vi "instrument final.vi"() -> ()   [LabVIEW 2019]
panel:
  out "Mesaj corupt":bool
  out "String 2":string
  in  "String":string
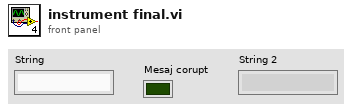
[diagram p1: front panel]
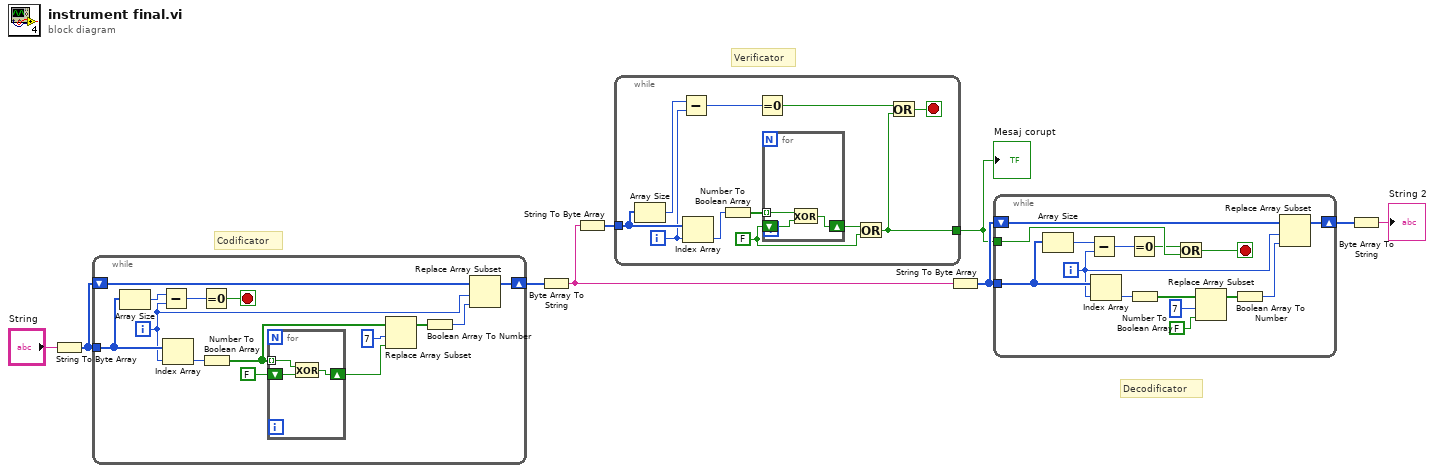
[diagram p0: block diagram]
diagram:
  # "Decodificator"
  # "Verificator"
  # "Codificator"
  n1 = String To Byte Array(string="String") -> (unsigned byte array=w5:u8[])
  n2 = while {
    tunnel: w5 -> [w23]
    shift-right: [w13] -> w4
    shift-left: w5 -> [w12]
    i -> [w11]
    stop <- w20 stop-if-true
    n3 = Array Size(array=w23) -> (size(s)=w22:i32)
    n4 = Subtract(x=w22, y=w11) -> (x-y=w21:i32)
    n5 = Index Array(array=w23, index=w11) -> (element=w15:u8)
    n6 = Equal To 0?(x=w21) -> (x = 0?=w20:bool)
    n7 = Number To Boolean Array(number=w15) -> (Boolean array=w17:bool[])
    n8 = for {
      tunnel: w17 -> [w24] mode=indexing
      shift-right: [w25] -> w18
      shift-left: FALSE -> [w26]
      n9 = Exclusive Or(1:w26, 2:w24) -> (0:w25:bool)
    }
    n10 = Replace Array Subset(array=w17, new element=w18, index=7) -> (w14:bool[])
    n11 = Boolean Array To Number(Boolean array=w14) -> (number=w10:u32)
    n12 = Replace Array Subset(array=w12, new element=w10, index=w11) -> (w13:u8[])
  }
  n13 = Byte Array To String(unsigned byte array=w4) -> (string=w2:string)
  n14 = String To Byte Array(string=w2) -> (unsigned byte array=w6:u8[])
  n15 = while {
    tunnel: w6 -> [w37]
    tunnel: [w27] -> w1
    i -> [w32]
    stop <- w28 stop-if-true
    w30 = FALSE
    n16 = Array Size(array=w37) -> (size(s)=w36:i32)
    n17 = Subtract(x=w36, y=w32) -> (x-y=w35:i32)
    n18 = Index Array(array=w37, index=w32) -> (element=w34:u8)
    n19 = Number To Boolean Array(number=w34) -> (Boolean array=w33:bool[])
    n20 = Equal To 0?(x=w35) -> (x = 0?=w29:bool)
    n21 = for {
      tunnel: w33 -> [w38] mode=indexing
      shift-right: [w39] -> w31
      shift-left: w30 -> [w40]
      n22 = Exclusive Or(1:w40, 2:w38) -> (0:w39:bool)
    }
    n23 = Or(x=w31, y=w30) -> (x .or. y?=w27:bool)
    n24 = Or(x=w29, y=w27) -> (x .or. y?=w28:bool)
  }
  "Mesaj corupt" <- w1
  n25 = String To Byte Array(string=w2) -> (unsigned byte array=w9:u8[])
  n26 = while {
    tunnel: w9 -> [w55]
    shift-right: [w49] -> w8
    shift-left: w9 -> [w48]
    tunnel: w1 -> [w42]
    i -> [w47]
    stop <- w43 stop-if-true
    n27 = Array Size(array=w55) -> (size(s)=w54:i32)
    n28 = Subtract(x=w54, y=w47) -> (x-y=w53:i32)
    n29 = Index Array(array=w55, index=w47) -> (element=w51:u8)
    n30 = Equal To 0?(x=w53) -> (x = 0?=w41:bool)
    n31 = Number To Boolean Array(number=w51) -> (Boolean array=w45:bool[])
    n32 = Or(x=w41, y=w42) -> (x .or. y?=w43:bool)
    n33 = Replace Array Subset(array=w45, new element=FALSE, index=7) -> (w50:bool[])
    n34 = Boolean Array To Number(Boolean array=w50) -> (number=w46:u32)
    n35 = Replace Array Subset(array=w48, new element=w46, index=w47) -> (w49:u8[])
  }
  n36 = Byte Array To String(unsigned byte array=w8) -> (string=→"String 2":string)
